vi "WLAN - TV - RW - ReadTestVectorFile(Rx) Dll.vi"(0 "Rx_TV_Path":string) -> (4 "PER Sweep Settings(Wfm * FreQ * Pwr)":T2[][][](array[typedef])=[[[{"Wfm_Index"=0, "Power Level Settings"={"Stop Power Level(dBm)"=-87.0, "Start Power Level(dBm)"=-67.0, "Step Size"=1.0}, "Carrier Frequency(Hz)"=2412000000.0, "# Freq Points"=4}], [{"Wfm_Index"=0, "Power Level Settings"={"Stop Power Level(dBm)"=-87.0, "Start Power Level(dBm)"=-67.0, "Step Size"=1.0}, "Carrier Frequency(Hz)"=5180000000.0, "# Freq Points"=4}], [{"Wfm_Index"=0, "Power Level Settings"={"Stop Power Level(dBm)"=-87.0, "Start Power Level(dBm)"=-67.0, "Step Size"=1.0}, "Carrier Frequency(Hz)"=5500000000.0, "# Freq Points"=4}], [{"Wfm_Index"=0, "Power Level Settings"={"Stop Power Level(dBm)"=-87.0, "Start Power Level(dBm)"=-67.0, "Step Size"=1.0}, "Carrier Frequency(Hz)"=5700000000.0, "# Freq Points"=4}]], [[{"Wfm_Index"=1, "Power Level Settings"={"Stop Power Level(dBm)"=-75.0, "Start Power Level(dBm)"=-55.0, "Step Size"=1.0}, "Carrier Frequency(Hz)"=2412000000.0, "# Freq Points"=4}], [{"Wfm_Index"=1, "Power Level Settings"={"Stop Power Level(dBm)"=-75.0, "Start Power Level(dBm)"=-55.0, "Step Size"=1.0}, "Carrier Frequency(Hz)"=5180000000.0, "# Freq Points"=4}], [{"Wfm_Index"=1, "Power Level Settings"={"Stop Power Level(dBm)"=-75.0, "Start Power Level(dBm)"=-55.0, "Step Size"=1.0}, "Carrier Frequency(Hz)"=5500000000.0, "# Freq Points"=4}], [{"Wfm_Index"=1, "Power Level Settings"={"Stop Power Level(dBm)"=-75.0, "Start Power Level(dBm)"=-55.0, "Step Size"=1.0}, "Carrier Frequency(Hz)"=5700000000.0, "# Freq Points"=4}]], [[{"Wfm_Index"=2, "Power Level Settings"={"Stop Power Level(dBm)"=-80.0, "Start Power Level(dBm)"=-60.0, "Step Size"=1.0}, "Carrier Frequency(Hz)"=2412000000.0, "# Freq Points"=4}], [{"Wfm_Index"=2, "Power Level Settings"={"Stop Power Level(dBm)"=-80.0, "Start Power Level(dBm)"=-60.0, "Step Size"=1.0}, "Carrier Frequency(Hz)"=5180000000.0, "# Freq Points"=4}], [{"Wfm_Index"=2, "Power Level Settings"={"Stop Power Level(dBm)"=-80.0, "Start Power Level(dBm)"=-60.0, "Step Size"=1.0}, "Carrier Frequency(Hz)"=5500000000.0, "# Freq Points"=4}], [{"Wfm_Index"=2, "Power Level Settings"={"Stop Power Level(dBm)"=-80.0, "Start Power Level(dBm)"=-60.0, "Step Size"=1.0}, "Carrier Frequency(Hz)"=5700000000.0, "# Freq Points"=4}]], [[{"Wfm_Index"=3, "Power Level Settings"={"Stop Power Level(dBm)"=-75.0, "Start Power Level(dBm)"=-55.0, "Step Size"=1.0}, "Carrier Frequency(Hz)"=2412000000.0, "# Freq Points"=4}], [{"Wfm_Index"=3, "Power Level Settings"={"Stop Power Level(dBm)"=-75.0, "Start Power Level(dBm)"=-55.0, "Step Size"=1.0}, "Carrier Frequency(Hz)"=5180000000.0, "# Freq Points"=4}], [{"Wfm_Index"=3, "Power Level Settings"={"Stop Power Level(dBm)"=-75.0, "Start Power Level(dBm)"=-55.0, "Step Size"=1.0}, "Carrier Frequency(Hz)"=5500000000.0, "# Freq Points"=4}], [{"Wfm_Index"=3, "Power Level Settings"={"Stop Power Level(dBm)"=-75.0, "Start Power Level(dBm)"=-55.0, "Step Size"=1.0}, "Carrier Frequency(Hz)"=5700000000.0, "# Freq Points"=4}]]], 6 "Waveform Generation Settings":T1[](array[typedef])=[{"Standard"=0, "Channel Bandwidth (Hz)"=20000000.0, "Idle Interval (s)"=0.0001, "MCS Index"=0, "80211n PLCP Frame Format"=0, "Payload Data Length (bytes)"=600, "OFDM Data Rate (Mbps)"=3, "DSSS Data Rate (Mbps)"=0, "Wfm_Index"=0}, {"Standard"=0, "Channel Bandwidth (Hz)"=20000000.0, "Idle Interval (s)"=0.0001, "MCS Index"=0, "80211n PLCP Frame Format"=0, "Payload Data Length (bytes)"=700, "OFDM Data Rate (Mbps)"=7, "DSSS Data Rate (Mbps)"=0, "Wfm_Index"=1}, {"Standard"=3, "Channel Bandwidth (Hz)"=20000000.0, "Idle Interval (s)"=0.0001, "MCS Index"=4, "80211n PLCP Frame Format"=0, "Payload Data Length (bytes)"=700, "OFDM Data Rate (Mbps)"=0, "DSSS Data Rate (Mbps)"=0, "Wfm_Index"=2}, {"Standard"=3, "Channel Bandwidth (Hz)"=20000000.0, "Idle Interval (s)"=0.0001, "MCS Index"=7, "80211n PLCP Frame Format"=0, "Payload Data Length (bytes)"=700, "OFDM Data Rate (Mbps)"=0, "DSSS Data Rate (Mbps)"=0, "Wfm_Index"=3}] {"DSSS Data Rate (Mbps)" items=["1", "2", "5.5 CCK", "5.5 PBCC", "11 CCK", "11 PBCC", "22", "33"]; "OFDM Data Rate (Mbps)" items=["6", "9", "12", "18", "24", "36", "48", "54"]; "80211n PLCP Frame Format" items=["Mixed Format", "Greenfield Format"]; "Standard" items=["80211A/G/J/P OFDM", "80211B/G DSSS", "80211G DSSSOFDM", "80211N MIMOOFDM", "80211AC MIMOOFDM"]}, 8 "#Packets":i32=100, 10 "PER Threshold":i32=10)   [LabVIEW 2011]
uses:
  Includes/WLAN - TV - RW - INC - Rx_PER_Sweep_Settings.ctl
  Includes/WLAN - TV - RW - INC - Rx_PER_Wfm_Settings.ctl
  <vilib>/Utility/file.llb/Read From Spreadsheet File (string).vi
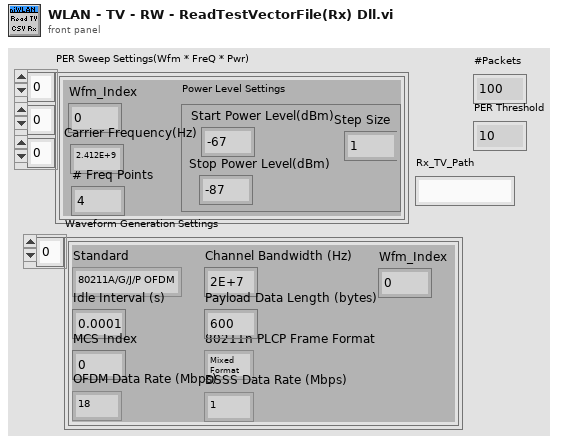
[diagram p1: front panel]
types:
  T1 = typedef "WLAN - TV - RW - INC - Rx_PER_Wfm_Settings.ctl" = cluster{"Standard":i32, "Channel Bandwidth (Hz)":dbl, "Idle Interval (s)":dbl, "MCS Index":i32, "80211n PLCP Frame Format":i32, "Payload Data Length (bytes)":i32, "OFDM Data Rate (Mbps)":i32, "DSSS Data Rate (Mbps)":i32, "Wfm_Index":i32}
  T2 = typedef "WLAN - TV - RW - INC - Rx_PER_Sweep_Settings.ctl" = cluster{"Wfm_Index":i32, "Power Level Settings":cluster{"Stop Power Level(dBm)":dbl, "Start Power Level(dBm)":dbl, "Step Size":dbl}, "Carrier Frequency(Hz)":dbl, "# Freq Points":i32}
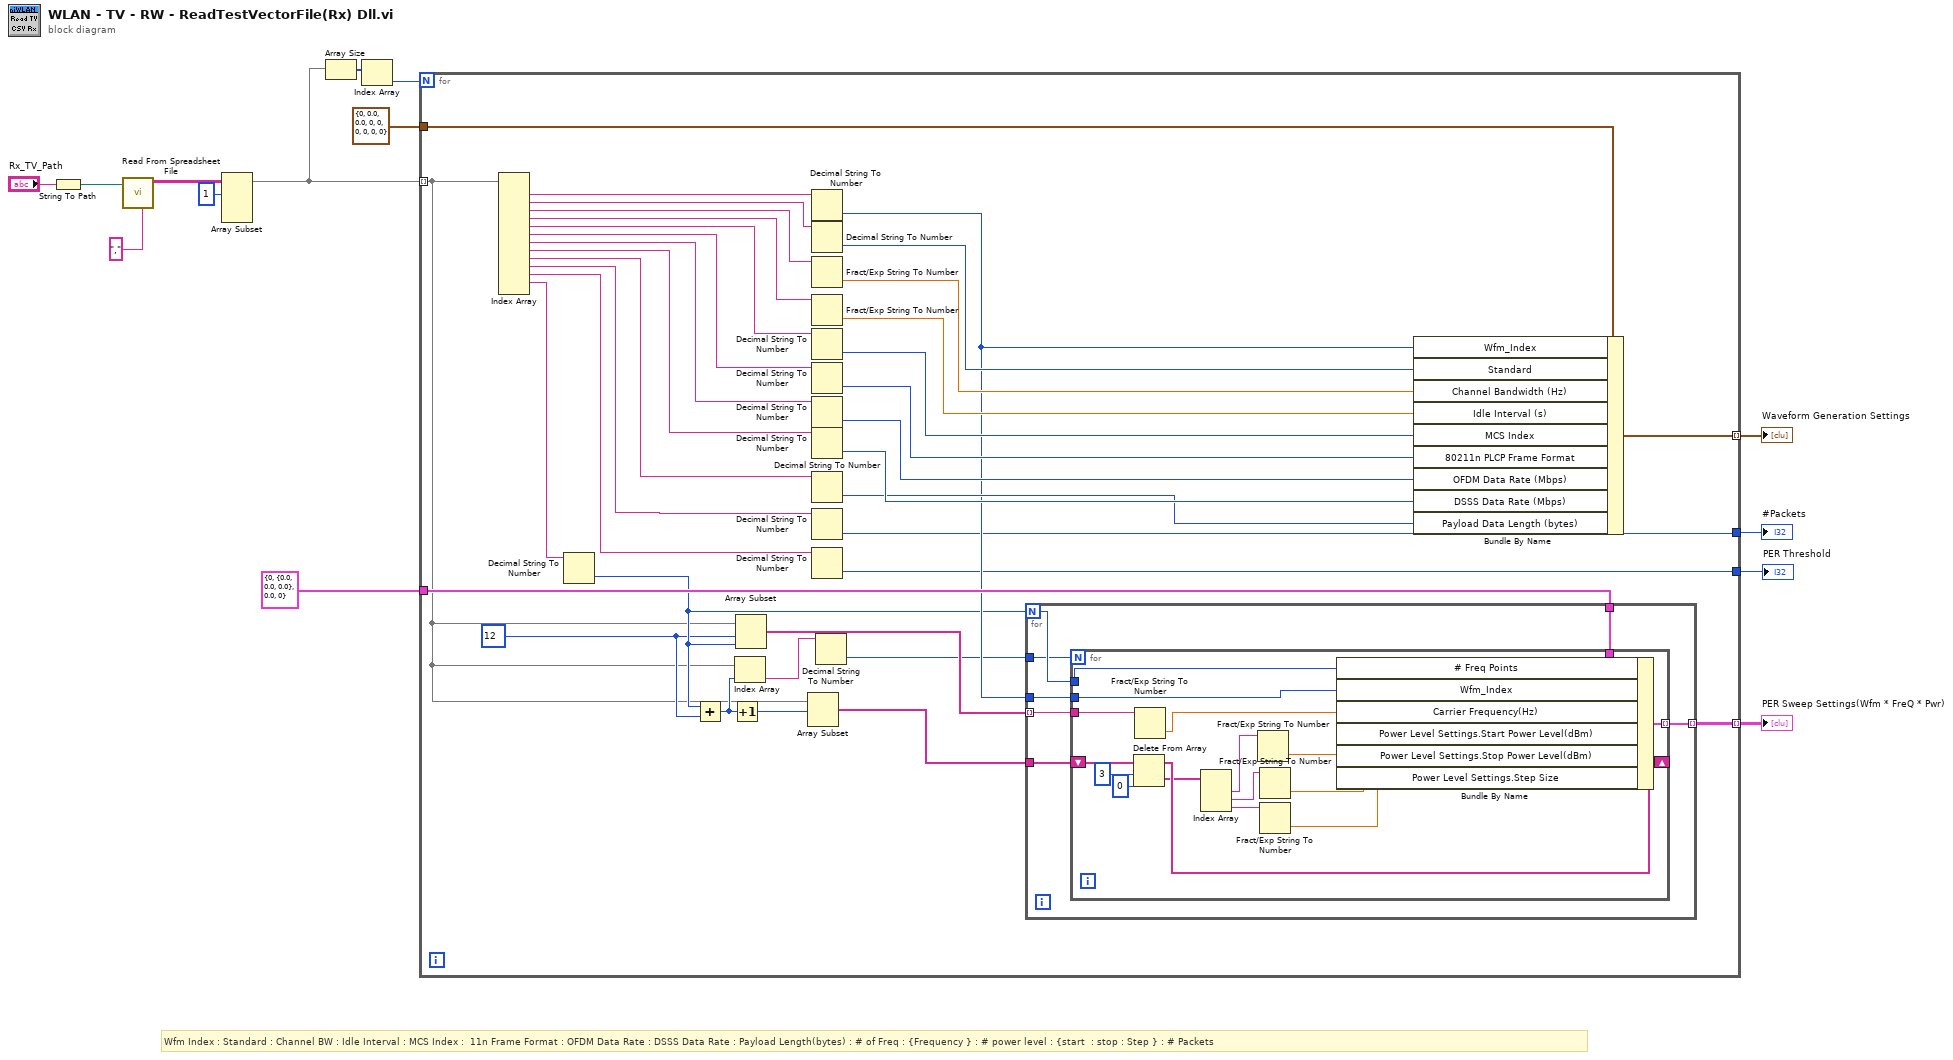
[diagram p0: block diagram]
diagram:
  # "Wfm Index : Standard : Channel BW : Idle Interval : MCS Index :  11n Frame Format : OFDM Data Rate : DSSS Data Rate : Payload Length(bytes) : # of Freq : {Frequency } : # power level : {start  : stop : Step } : # Packets"
  n1 = String To Path(string="Rx_TV_Path") -> (path=w2:path)
  n2 = call-poly <vilib>:"Read From Spreadsheet File.vi"("delimiter (\\t)"="," ("delimiter (\\t)"), "file path (dialog if empty)"=w2) -> ("all rows"=w5:string[][])  [unwired: 5 in, 4 out]
  n3 = Array Subset(array=w5, index (row)=1 ("index")) -> (w6:string[][])  [unwired: 3 in]
  n4 = Array Size(array=w6) -> (size(s)=w13:i32[])
  n5 = Index Array(array=w13) -> (element=w12:i32)  [unwired: 1 in]
  n6 = for {
    N: w12 -> [_]
    tunnel: w6 -> [w20] mode=indexing
    tunnel: T2 {"Wfm_Index"=0, "Power Level Settings"={"Stop Power Level(dBm)"=0.0, "Start Power Level(dBm)"=0.0, "Step Size"=0.0}, "Carrier Frequency(Hz)"=0.0, "# Freq Points"=0} ("Sweep Settings") -> [w31]
    tunnel: T1 {"Standard"=0, "Channel Bandwidth (Hz)"=0.0, "Idle Interval (s)"=0.0, "MCS Index"=0, "80211n PLCP Frame Format"=0, "Payload Data Length (bytes)"=0, "OFDM Data Rate (Mbps)"=0, "DSSS Data Rate (Mbps)"=0, "Wfm_Index"=0} ("Rx Measurements Settings") -> [w49]
    tunnel: [w32] -> w9 mode=indexing
    tunnel: [w30] -> w8 mode=indexing
    tunnel: [w18] -> w7
    tunnel: [w15] -> w3
    w26 = 12 ("index")
    n7 = Index Array(array=w20) -> (element #1=w50:string, element #2=w48:string, element #3=w47:string, element #4=w46:string, element #5=w45:string, element #6=w44:string, element #7=w43:string, element #8=w42:string, element #9=w41:string, element #10=w19:string, element #11=w16:string, element #12=w17:string)  [unwired: 13 in, 1 out]
    n8 = Decimal String To Number(string=w17) -> (number=w27:i32)  [unwired: 2 in, 1 out]
    n9 = Add(x=w27, y=w26) -> (x+y=w25:i32)
    n10 = Increment(x=w25) -> (x+1=w21:i32)
    n11 = Index Array(array=w20, index=w25) -> (element=w24:string)
    n12 = Array Subset(array=w20, index=w26, length=w27) -> (w29:string[])
    n13 = Array Subset(array=w20, index=w21) -> (w23:string[])  [unwired: 1 in]
    n14 = Decimal String To Number(string=w50) -> (number=w28:i32)  [unwired: 2 in, 1 out]
    n15 = Decimal String To Number(string=w48) -> (number=w40:i32)  [unwired: 2 in, 1 out]
    n16 = Fract/Exp String To Number(string=w47) -> (number=w39:dbl)  [unwired: 3 in, 1 out]
    n17 = Fract/Exp String To Number(string=w46) -> (number=w38:dbl)  [unwired: 3 in, 1 out]
    n18 = Decimal String To Number(string=w45) -> (number=w37:i32)  [unwired: 2 in, 1 out]
    n19 = Decimal String To Number(string=w44) -> (number=w36:i32)  [unwired: 2 in, 1 out]
    n20 = Decimal String To Number(string=w43) -> (number=w35:i32)  [unwired: 2 in, 1 out]
    n21 = Decimal String To Number(string=w42) -> (number=w34:i32)  [unwired: 2 in, 1 out]
    n22 = Decimal String To Number(string=w41) -> (number=w33:i32)  [unwired: 2 in, 1 out]
    n23 = Decimal String To Number(string=w19) -> (number=w18:i32)  [unwired: 2 in, 1 out]
    n24 = Decimal String To Number(string=w16) -> (number=w15:i32)  [unwired: 2 in, 1 out]
    n25 = Decimal String To Number(string=w24) -> (number=w22:i32)  [unwired: 2 in, 1 out]
    n26 = for {
      N: w27 -> [w53]
      tunnel: w29 -> [w57] mode=indexing
      tunnel: w28 -> [w56]
      tunnel: w31 -> [w55]
      tunnel: [w54] -> w30 mode=indexing
      tunnel: w22 -> [w52]
      tunnel: w23 -> [w51]
      n27 = for {
        N: w52 -> [_]
        tunnel: w57 -> [w70]
        tunnel: w56 -> [w73]
        tunnel: w55 -> [w74]
        tunnel: [w72] -> w54 mode=indexing
        tunnel: w53 -> [w71]
        shift-right: [w65] -> _
        shift-left: w51 -> [w68]
        n28 = Delete From Array(array=w68, length=3, index=0) -> (deleted portion=w64:string[], array with subset deleted=w65:string[])
        n29 = Fract/Exp String To Number(string=w70) -> (number=w69:dbl)  [unwired: 3 in, 1 out]
        n30 = Index Array(array=w64) -> (element #1=w63:string, element #2=w62:string, element #3=w61:string)  [unwired: 3 in]
        n31 = Fract/Exp String To Number(string=w63) -> (number=w58:dbl)  [unwired: 3 in, 1 out]
        n32 = Fract/Exp String To Number(string=w62) -> (number=w59:dbl)  [unwired: 3 in, 1 out]
        n33 = Fract/Exp String To Number(string=w61) -> (number=w60:dbl)  [unwired: 3 in, 1 out]
        n34 = Bundle By Name(cluster=w74, "# Freq Points"=w71, "Wfm_Index"=w73, "Carrier Frequency(Hz)"=w69, "Power Level Settings.Start Power Level(dBm)"=w58, "Power Level Settings.Stop Power Level(dBm)"=w59, "Power Level Settings.Step Size"=w60) -> (w72:T2)
      }
    }
    n35 = Bundle By Name(cluster=w49, "Wfm_Index"=w28, "Standard"=w40, "Channel Bandwidth (Hz)"=w39, "Idle Interval (s)"=w38, "MCS Index"=w37, "80211n PLCP Frame Format"=w36, "OFDM Data Rate (Mbps)"=w35, "DSSS Data Rate (Mbps)"=w34, "Payload Data Length (bytes)"=w33) -> (w32:T1)
  }
  "PER Sweep Settings(Wfm * FreQ * Pwr)" <- w8
  "Waveform Generation Settings" <- w9
  "#Packets" <- w7
  "PER Threshold" <- w3
